vi "Alicat Simplified Driver Example_Logging.vi"() -> ()   [LabVIEW 2020]
doc: "Simplified example program for initializing the COM port, determining the data frame of an Alicat, acquiring the data of the same Alicat, and logging desired variables to a text file. \n\nThis is a slightly more feature rich version of the Alicat Simplified Driver Example, and contains an example of a method for implementing fast, selective data logging."
panel:
  out "Measurement Data":T1
  in  "Data Logging Options (If valid)":T2={"Absolute Press."=TRUE, "Gauge/Diff. Press."=TRUE, "Barometric Press."=TRUE, "Temperature"=TRUE, "Volumetric"=TRUE, "Mass Flow"=TRUE, "Setpoint"=TRUE, "Valve Drive"=FALSE, "Totalizer"=TRUE, "Tot. Timer [s]"=FALSE, "Tot. Avg. Flow"=FALSE, "Tot. Peak Flow"=FALSE, "Gas Selected"=TRUE, "Log Data"=TRUE}
  in  "Minimum time between \nreadings [ms]":u32
  out "Measurements\nper second":dbl
  out "Elapsed Time [ms]":dbl caption="Elapsed Time (s)"
  in  "End Program":bool
  out "Error Text":string
  out "Error Present":bool
  out "Range Exceeded":bool
  in  "COM Port Settings":T3={"Unit ID"="A", "Baud Rate"=enum."19200", "VISA Sesssion In"="COM1"}
  # "Totalizer Timer"
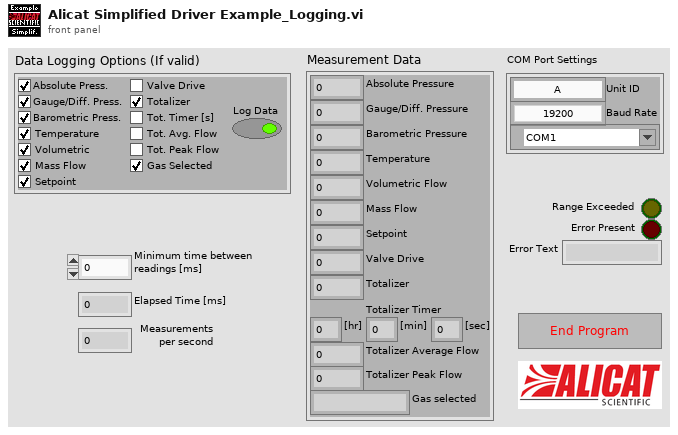
[diagram p1: front panel]
types:
  T1 = cluster{"Absolute Pressure":dbl, "Gauge/Diff. Pressure":dbl, "Barometric Pressure":dbl, "Temperature":dbl, "Volumetric Flow":dbl, "Mass Flow":dbl, "Setpoint":dbl, "Valve Drive":dbl, "Totalizer":dbl, "[hr]":dbl, "[min]":dbl, "[sec]":dbl, "Totalizer Average Flow":dbl, "Totalizer Peak Flow":dbl, "Gas selected":string}
  T2 = cluster{"Absolute Press.":bool, "Gauge/Diff. Press.":bool, "Barometric Press.":bool, "Temperature":bool, "Volumetric":bool, "Mass Flow":bool, "Setpoint":bool, "Valve Drive":bool, "Totalizer":bool, "Tot. Timer [s]":bool, "Tot. Avg. Flow":bool, "Tot. Peak Flow":bool, "Gas Selected":bool, "Log Data":bool}
  T3 = cluster{"Unit ID":string, "Baud Rate":enum8{"2400", "9600", "19200", "38400", "57600", "115200", "Unknown"}, "VISA Sesssion In":refnum<visa-resource-name>}
  T4 = enum16{"open", "replace", "create", "open or create", "replace or create", "replace or create with confirmation"}
  T5 = typedef "Data Frame.ctl" = cluster{"Absolute Pressure":bool, "Gauge/Diff. Pressure":bool, "Barometric Pressure":bool, "Temperature":bool, "Volumetric":bool, "Mass":bool, "Setpoint":bool, "Valve Drive":bool, "Totalizer":bool, "Totalizer Timer":bool, "Totalizer Average Flow":bool, "Totalizer Peak Flow":bool, "Gas Selected":bool, "Tot. Timer Format":u16}
  T6 = typedef "Data Cluster.ctl" = cluster{"Absolute Pressure":dbl, "Gauge/Diff. Pressure":dbl, "Barometric Pressure":dbl, "Temperature":dbl, "Volumetric Flow":dbl, "Mass Flow":dbl, "Setpoint":dbl, "Valve Drive":dbl, "Totalizer":dbl, "[hr]":dbl, "[min]":dbl, "[sec]":dbl, "Totalizer Average Flow":dbl, "Totalizer Peak Flow":dbl, "Gas selected":string}
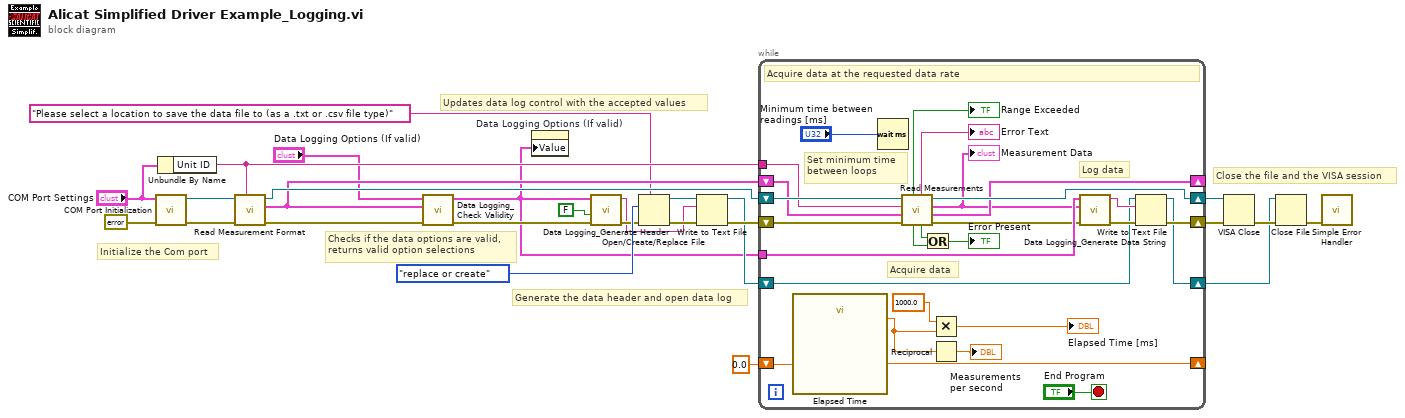
[diagram p0: block diagram]
diagram:
  # "Updates data log control with the accepted values"
  # "Checks if the data options are valid,\nreturns valid option selections"
  # "Generate the data header and open data log"
  # "Close the file and the VISA session"
  # "Initialize the Com port"
  n1 = call "COM Port Initialization.vi"("error in (no error)"=errorcluster {"status"=FALSE, "code"=0, "source"=""}, "Communication Settings"="COM Port Settings") -> ("error out"=w22:errorcluster, "VISA Session Out"=w21:refnum<visa-resource-name>)  [unwired: 8 in]
  n2 = Unbundle By Name("COM Port Settings") -> ("Unit ID"=w19:string)
  n3 = call "Read Measurement Format.vi"("Unit ID (A)"=w19, "error in"=w22, "VISA Session In"=w21) -> ("error out"=w10:errorcluster, "Data Frame Format"=w18:T5, "VISA Session Out"=w20:refnum<visa-resource-name>)  [unwired: 6 in]
  n4 = call "Data Logging_Check Validity.vi"("error in"=w10, "Data Frame Format"=w18, "Data Logging Options (If valid)"="Data Logging Options (If valid)") -> ("error out"=w16:errorcluster, "Validated Logging Options"=w2:T2)  [unwired: 6 in, 1 out]
  n5 = property on="Data Logging Options (If valid)" class="Clust (strict)"("Value"=w2) -> ()  [unwired: 2 in, 2 out]
  n6 = call "Data Logging_Generate Header.vi"("error in"=w16, "Include Units\nin Header (F)"=FALSE ("Include Units\nin Header (default is F)"), "Data Logging Options"=w2) -> ("error out"=w12:errorcluster, "Data Log Header"=w8:string)  [unwired: 6 in, 1 out]
  n7 = Open/Create/Replace File(error in=w12, prompt="Please select a location to save the data file to (as a .txt or .csv file type)", operation (0:open)=T4."replace or create") -> (refnum out=w15:refnum<file>, error out=w14:errorcluster)  [unwired: 3 in, 1 out]
  n8 = Write to Text File(file (use dialog)=w15, text=w8, error in=w14) -> (refnum out=w7:refnum<file>, error out=w11:errorcluster)  [unwired: 1 in, 1 out]
  n9 = while {
    shift-right: [w50] -> _
    shift-left: 0.0 ("Set Start Time (s)") -> [w53]
    shift-right: [w30] -> w6
    shift-left: w11 -> [w52]
    shift-right: [w49] -> w23
    shift-left: w20 -> [w51]
    tunnel: w19 -> [w48]
    shift-right: [w42] -> _
    shift-left: w18 -> [w47]
    shift-right: [w28] -> w3
    shift-left: w7 -> [w29]
    tunnel: w2 -> [w34]
    stop <- "End Program" stop-if-true
    # "Log data"
    # "Set minimum time\nbetween loops"
    # "Acquire data"
    # "Acquire data at the requested data rate"
    n10 = call "Elapsed Time"("Set Start Time (s)"=w53) -> ("Get Start Time (s)"=w50:dbl, "Elapsed Time (s)"=w36:dbl)  [unwired: 11 in, 6 out]
    n11 = Wait (ms)(milliseconds to wait="Minimum time between \nreadings [ms]") -> ()  [unwired: 1 out]
    n12 = call "Read Measurements.vi"("error in"=w52, "Data Frame Format In"=w47, "Unit ID (A)"=w48, "VISA Session In"=w51) -> ("error out"=w33:errorcluster, "Data Frame Format Out"=w42:T5, "Data Cluster"=w27:T6, "VISA Session Out"=w49:refnum<visa-resource-name>, "Unknown Dataframe Info"=w46:bool, "Error/Overrange/Unknown String"=→"Error Text":string, "Error Present"=w45:bool, "Range Exceeded"=→"Range Exceeded":bool)
    "Measurement Data" <- w27
    n13 = Or(x=w46, y=w45) -> (x .or. y?=→"Error Present":bool)
    n14 = Multiply(x=1000.0 ("y"), y=w36) -> (x*y=→"Elapsed Time [ms]":dbl)
    n15 = Reciprocal(x=w36) -> (1/x=→"Measurements\nper second":dbl)
    n16 = call "Data Logging_Generate Data String.vi"("error in"=w33, "Measurement Data"=w27, "Data Logging Options"=w34) -> ("error out"=w32:errorcluster, "Data Log String"=w31:string)  [unwired: 6 in, 1 out]
    n17 = Write to Text File(file (use dialog)=w29, text=w31, error in=w32) -> (refnum out=w28:refnum<file>, error out=w30:errorcluster)  [unwired: 1 in, 1 out]
  }
  n18 = VISA Close(VISA resource name=w23, error in (no error)=w6) -> (error out=w5:errorcluster)
  n19 = Close File(refnum=w3, error in=w5) -> (error out=w4:errorcluster)  [unwired: 1 out]
  n20 = call <vilib>:"Simple Error Handler.vi"("error in (no error)"=w4) -> ()  [unwired: 4 in, 5 out]
